vi "Set Delay.vi"(8 "error in (no error)":errorcluster, 9 "Rate (ps/s)":dbl, 10 "Delay (ps)":dbl, 11 "Instrument.Delay in":refnum<class "Instrument.OpticalDelayLine.lvclass">) -> (0 "error out":errorcluster, 3 "Instrument.Delay out":refnum<class "Instrument.OpticalDelayLine.lvclass">)   [LabVIEW 2020, in "Instrument.OpticalDelayLine.lvclass"]
uses:
  Instrument.OpticalDelayLine.lvclass
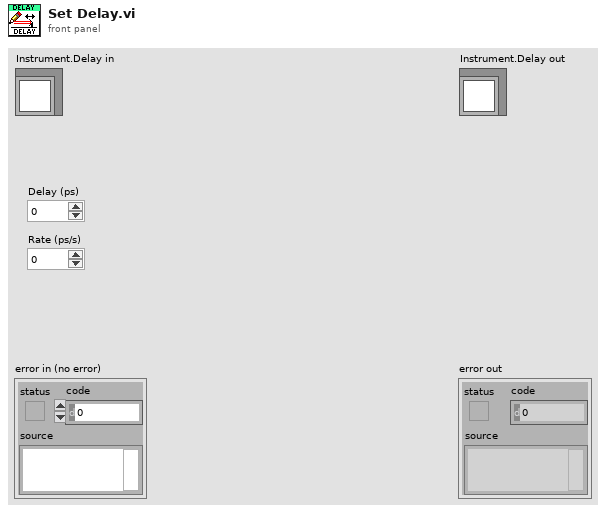
[diagram p1: front panel]
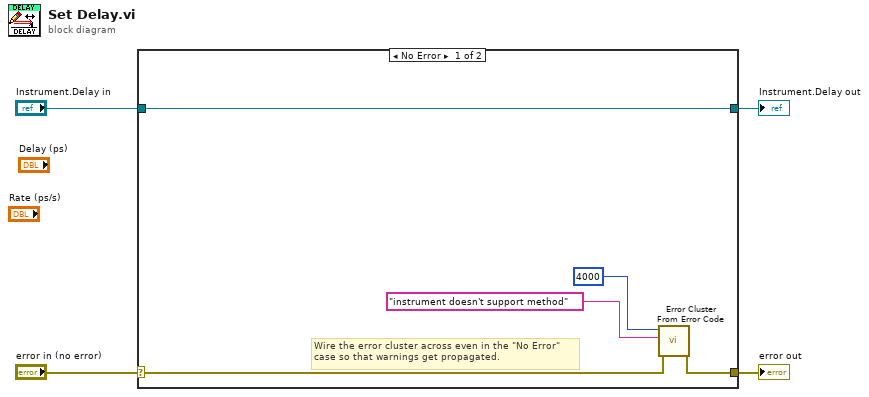
[diagram p0: block diagram]
diagram:
  n1 = case shown="No Error" "error in (no error)" {
    selector: "error in (no error)" -> [w6 w11]
    tunnel: [w5 w11] -> w3
    tunnel: [w9 w10] -> w1
    tunnel: "Instrument.Delay in" -> [w9 w10]
    frame No Error {
      # "Wire the error cluster across even in the \"No Error\"\ncase so that warnings get propagated."
      n2 = call <vilib>:"Error Cluster From Error Code.vi"("error in (no error)"=w6, "error message (\"\")"="instrument doesn't support method" ("error message (\"\")"), "error code (0)"=4000) -> ("error out"=w5:errorcluster)  [unwired: 6 in]
    }
    frame Error {
    }
  }
  "error out" <- w3
  "Instrument.Delay out" <- w1
